vi "NS_ReadWriteAttribute_IPE.vi"(0 "object in":refnum<class "NativeSubTemplate_4x4x4.lvclass">, 5 "error in (no error)":errorcluster) -> (14 "object out":refnum<class "NativeSubTemplate_4x4x4.lvclass">, 19 "error out":errorcluster)   [LabVIEW 2020, in "NativeSubTemplate_4x4x4.lvclass"]
uses:
  <resource>/Framework/Providers/Open_GDS/ClassProviders/Provider_LvNativeClass/Templates/NativeSubTemplate_4x4x4/NativeSubTemplate_4x4x4.lvclass
  <resource>/Framework/Providers/Open_GDS/ClassProviders/Provider_LvNativeClass/Templates/NativeSubTemplate_4x4x4/NativeSubTemplate_4x4x4.lvclass/NativeSubTemplate_4x4x4.ctl
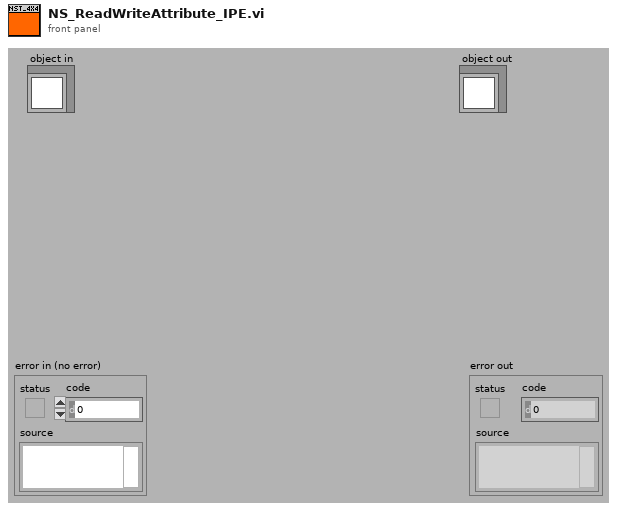
[diagram p1: front panel]
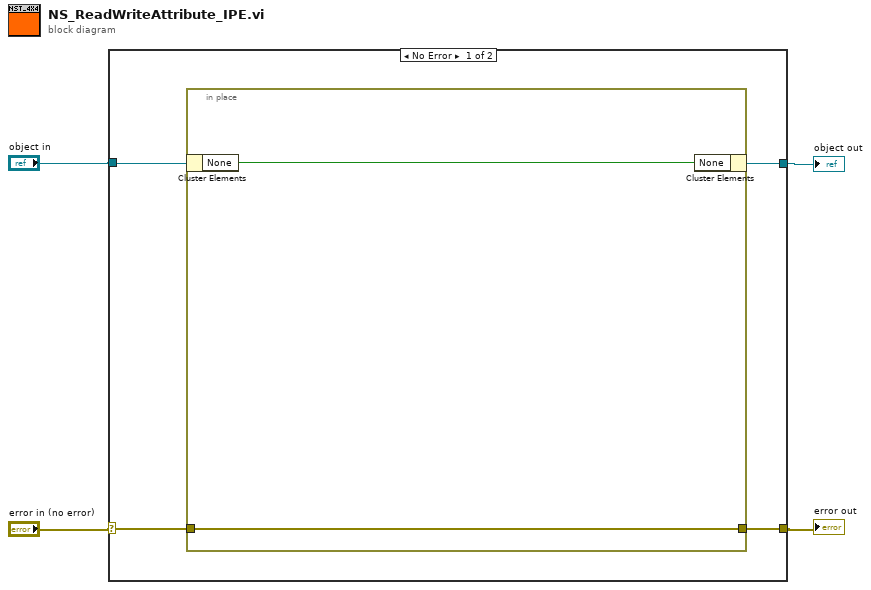
[diagram p0: block diagram]
diagram:
  n1 = case shown="No Error" "error in (no error)" {
    selector: "error in (no error)" -> [w5 w12]
    tunnel: [w6 w12] -> w1
    tunnel: [w7 w11] -> w2
    tunnel: "object in" -> [w8 w11]
    frame No Error {
      n2 = in-place {
        in-place-border: [w9] -> w6
        in-place-border: w5 -> [w9]
        n3 = in-place-cluster #1(w8) -> ("None"=w10:bool)
        n4 = in-place-cluster #1("None"=w10) -> (w7:refnum<class "NativeSubTemplate_4x4x4.lvclass">)
      }
    }
    frame Error {
    }
  }
  "error out" <- w1
  "object out" <- w2
